vi "System Identification.vi"() -> ()   [LabVIEW 2019]
doc: "This example demonstrates how to apply an LMS adaptive filter to system identification applications. This example uses a lowpass FIR filter to simulate an unknown system. The input to the unknown system is Gaussian white noise. Use the input to the unknown system as the input to the adaptive filter. Use the output from the unknown system as the reference of the adaptive filter. The coefficients of the adaptive filter converge to the coefficients of the unknown system when the adaptive filter converges. \n\nRun this VI and observe how the coefficients of the adaptive filter converge to those of the unknown system."
uses:
  <vilib>/addons/Adaptive Filters/Create/AFT Create FIR LMS (Real).vi
  <vilib>/addons/Adaptive Filters/Processing/AFT Filter Signal and Update Coefficients (Real, PtByPt).vi
  <vilib>/addons/Adaptive Filters/Analysis/AFT Get Coefficients (FIR, Real).vi
  <vilib>/addons/Adaptive Filters/NI_AdaptiveFilter.lvlib
panel:
  in  "Tab Control":enum32{"Background", "System Identification"}(tab)
  in  "Step Size":dbl=0.002 min=0.0 step=0.01
  in  "Filter Length":i32=25 min=2
  out "Coefficients":dbl[][](graph)
  out "Error Signal":dbl(graph)
  in  "stop":bool
  # "Refer to the System Identification topic in the LabVIEW Help for more information about the background of system identification. \nSelect Help>>Show Context Help and move the cursor over the VI icon of this example for more information."
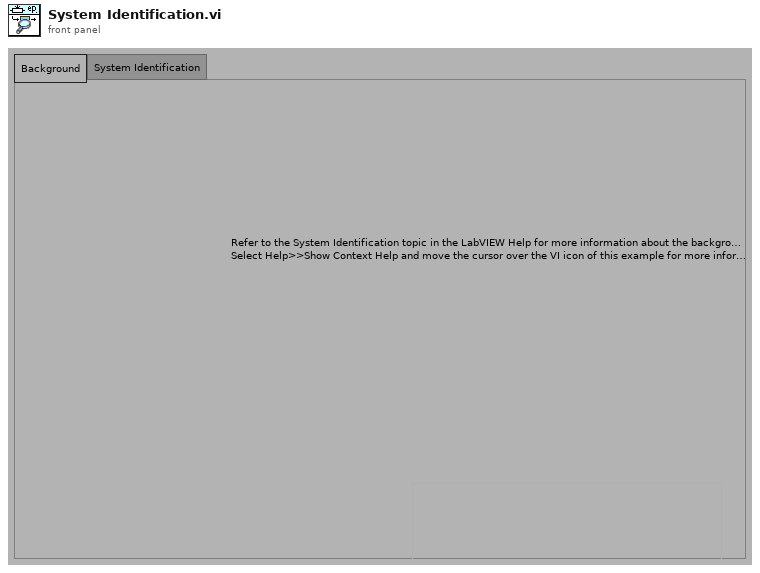
[diagram p1: front panel]
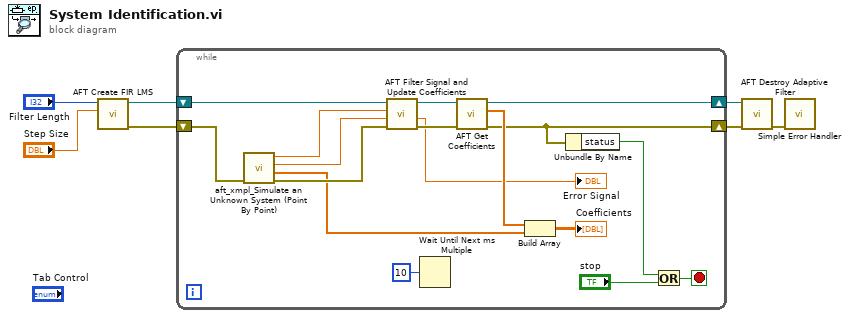
[diagram p0: block diagram]
diagram:
  n1 = call-poly <vilib>:"AFT Create FIR LMS.vi"("step size"="Step Size", "filter length"="Filter Length") -> ("error out"=w5:errorcluster, "adaptive filter out"=w6:refnum<k20>)  [unwired: 2 in, 6 out]
  n2 = while {
    shift-right: [w22] -> w4
    shift-left: w6 -> [w23]
    shift-right: [w11] -> w3
    shift-left: w5 -> [w12]
    stop <- w9 stop-if-true
    n3 = call "aft_xmpl_Simulate an Unknown System (Point By Point).vi"("error in (no error)"=w12) -> ("error out"=w24:errorcluster, "unknown system coefficients"=w13:dbl[], "response signal"=w14:dbl, "stimulus signal"=w15:dbl)  [unwired: 7 out]
    n4 = call-poly <vilib>:"AFT Filter Signal and Update Coefficients.vi"("error in (no error)"=w24, "d(n)"=w14, "x(n)"=w15, "adaptive filter in"=w23) -> ("error out"=w20:errorcluster, "e(n)"=→"Error Signal":dbl, "adaptive filter out"=w21:refnum<k20>)  [unwired: 2 in, 3 out]
    n5 = Wait Until Next ms Multiple(millisecond multiple=u32 10) -> ()  [unwired: 1 out]
    n6 = call-poly <vilib>:"AFT Get Coefficients.vi"("error in (no error)"=w20, "adaptive filter in"=w21) -> ("error out"=w11:errorcluster, "coefficients"=w19:dbl[], "adaptive filter out"=w22:refnum<k20>)  [unwired: 7 out]
    n7 = Build Array(w19, w13) -> (→"Coefficients":dbl[][])
    n8 = Unbundle By Name(w11) -> ("status"=w8:bool)
    n9 = Or(x=w8, y="stop") -> (x .or. y?=w9:bool)
  }
  n10 = call <vilib>:"AFT Destroy Adaptive Filter.vi"("error in (no error)"=w3, "adaptive filter in"=w4) -> ("error out"=w1:errorcluster)  [unwired: 9 out]
  n11 = call <vilib>:"Simple Error Handler.vi"("error in (no error)"=w1) -> ()  [unwired: 1 in, 8 out]
